vi "Destructor.vi"(8 "error in":errorcluster, 11 "Document in":refnum<class "Document.lvclass">) -> (0 "error out":errorcluster)   [LabVIEW 2021, in "ProligentXMLGenerator.lvlib" / "Document.lvclass"]
uses:
  Document.lvclass
  Document.lvclass/Document.ctl
  CustomData/CustomData.lvclass
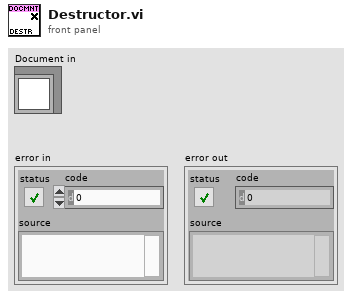
[diagram p1: front panel]
types:
  T1 = typedef "ProligentXMLGenerator.lvlib/Document.lvclass/Data.ctl" = cluster{"Name":string, "CustomData":refnum<class "CustomData.lvclass">, "Identifier":refnum<class "Guid.lvclass">, "NameType":refnum<class "NonEmptyString_255.lvclass">, "FileName":refnum<class "NonEmptyString_255.lvclass">, "Description":refnum<class "NonNullableString_600.lvclass">, "FilePath":path, "DestinationFolder":path}
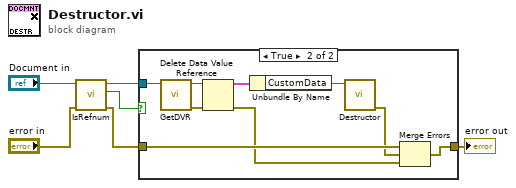
[diagram p0: block diagram]
diagram:
  n1 = call "IsRefnum.vi"("error in"="error in", "Document in"="Document in") -> ("error out"=w1:errorcluster, "IsRefnum"=w3:bool, "Document out"=w4:refnum<class "Document.lvclass">)  [unwired: 7 in]
  n2 = case shown="True" w3 {
    tunnel: w1 -> [w7 w16]
    tunnel: [w7 w15] -> w6
    tunnel: w4 -> [_ w12]
    frame False {
    }
    frame True {
      n3 = call "GetDVR.vi"("Document in"=w12) -> ("error out"=w13:errorcluster, "DVRReference"=w14:refnum<data-value>)  [unwired: 9 in]
      n4 = Delete Data Value Reference(data value reference=w14, error in=w13) -> (data value=w10:T1, error out=w11:errorcluster)
      n5 = Unbundle By Name(w10) -> ("CustomData"=w9:refnum<class "CustomData.lvclass">)
      n6 = call "Destructor.vi"("CustomDataType"=w9) -> ("error out"=w8:errorcluster)  [unwired: 10 in]
      n7 = Merge Errors(w16, w8, w11) -> (w15:errorcluster)
    }
  }
  "error out" <- w6
